vi "SV Peak Levels (N Ch).vi"(7 "reset":bool, 11 "input signals":waveform(dbl)[](array[waveform])) -> (0 "minima":dbl[](array[numeric]), 1 "maxima":dbl[](array[numeric]), 2 "max-min levels":dbl[](array[numeric]), 3 "peak levels":dbl[](array[numeric]), 4 "durations (s)":dbl[](array[numeric]), 5 "timestamps":timestamp[](array[timestamp]))   [LabVIEW 2017]
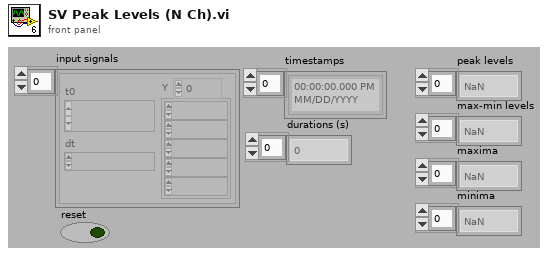
[diagram p1: front panel]
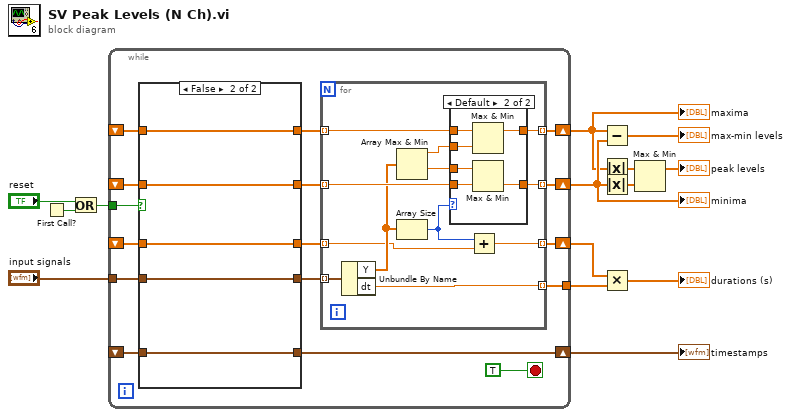
[diagram p0: block diagram]
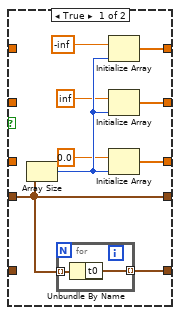
[diagram p2: hidden frame]
diagram:
  n1 = First Call?() -> (First Call?: T/F=w5:bool)
  n2 = Or(x="reset", y=w5) -> (x .or. y?=w3:bool)
  n3 = while {
    tunnel: w3 -> [w25]
    shift-right: [w29] -> w1
    shift-left: _ -> [w22]
    shift-right: [w30] -> w2
    shift-left: _ -> [w21]
    shift-right: [w28] -> w7
    shift-left: _ -> [w20]
    tunnel: "input signals" -> [w24]
    shift-right: [w16] -> w9
    shift-left: _ -> [w15]
    tunnel: [w26] -> w8
    stop <- TRUE stop-if-true
    n4 = case shown="False" w25 {
      tunnel: w21 -> [_ w45]
      tunnel: w22 -> [_ w46]
      tunnel: [w35 w46] -> w17
      tunnel: [w34 w45] -> w18
      tunnel: [w33 w44] -> w19
      tunnel: w20 -> [_ w44]
      tunnel: w24 -> [w32 w42]
      tunnel: [w32 w42] -> w23
      tunnel: [w31 w43] -> w16
      tunnel: w15 -> [_ w43]
      frame True {
        n5 = Array Size(array=w32) -> (size(s)=w39:i32)
        n6 = for {
          tunnel: w32 -> [w41] mode=indexing
          tunnel: [w40] -> w31 mode=indexing
          n7 = Unbundle By Name(w41) -> ("t0"=w40:timestamp)
        }
        n8 = Initialize Array(-inf ("t"), w39) -> (w35:dbl[])
        n9 = Initialize Array(inf ("t"), w39) -> (w34:dbl[])
        n10 = Initialize Array(0.0, w39) -> (w33:dbl[])
      }
      frame False {
      }
    }
    n11 = for {
      tunnel: [w58] -> w30 mode=indexing
      tunnel: [w57] -> w29 mode=indexing
      tunnel: [w47] -> w28 mode=indexing
      tunnel: w23 -> [w56] mode=indexing
      tunnel: w18 -> [w53] mode=indexing
      tunnel: w17 -> [w54] mode=indexing
      tunnel: [w55] -> w26 mode=indexing
      tunnel: w19 -> [w49] mode=indexing
      n12 = Unbundle By Name(w56) -> ("Y"=w52:dbl[], "dt"=w55:dbl)
      n13 = Array Max & Min(array=w52) -> (max value=w51:dbl, min value=w50:dbl)  [unwired: 2 out]
      n14 = Array Size(array=w52) -> (size(s)=w48:i32)
      n15 = case shown="Default" w48 {
        tunnel: w54 -> [w60 w64]
        tunnel: w53 -> [w59 w63]
        tunnel: [w59 w66] -> w58
        tunnel: [w60 w65] -> w57
        tunnel: w51 -> [_ w62]
        tunnel: w50 -> [_ w61]
        frame 0 {
        }
        frame Default {
          n16 = Max & Min(x=w64, y=w62) -> (max(x,y)=w65:dbl)  [unwired: 1 out]
          n17 = Max & Min(x=w61, y=w63) -> (min(x,y)=w66:dbl)  [unwired: 1 out]
        }
      }
      n18 = Add(x=w48, y=w49) -> (x+y=w47:dbl)
    }
  }
  "timestamps" <- w9
  "maxima" <- w1
  "minima" <- w2
  n19 = Subtract(x=w1, y=w2) -> (x-y=→"max-min levels":dbl[])
  n20 = Absolute Value(x=w1) -> (abs(x)=w13:dbl[])
  n21 = Absolute Value(x=w2) -> (abs(x)=w12:dbl[])
  n22 = Multiply(x=w7, y=w8) -> (x*y=→"durations (s)":dbl[])
  n23 = Max & Min(x=w13, y=w12) -> (max(x,y)=→"peak levels":dbl[])  [unwired: 1 out]
